vi "3 Mirrors Convert to Volts.vi"(0 "Global Rectangle":i32[](array[numeric]), 2 "Scan Freq (Hz)":dbl, 5 "X Center":dbl, 7 "Y Center":dbl, 9 "M1 Volts Per Px":dbl, 11 "M2 Volts Per Px":dbl) -> (8 "Voltage Data":T1)   [LabVIEW 2020]
uses:
  3 Mirror Scan Type Defs/3 Mirror Scan ROI Voltage Data.ctl
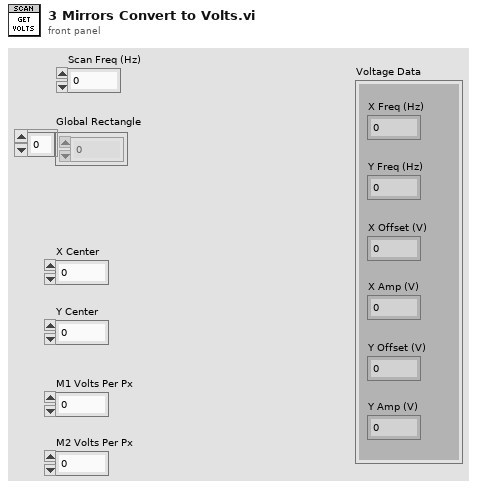
[diagram p1: front panel]
types:
  T1 = typedef "3 Mirror Scan ROI Voltage Data.ctl" = cluster{"X Freq (Hz)":dbl, "Y Freq (Hz)":dbl, "X Offset (V)":dbl, "X Amp (V)":dbl, "Y Offset (V)":dbl, "Y Amp (V)":dbl}
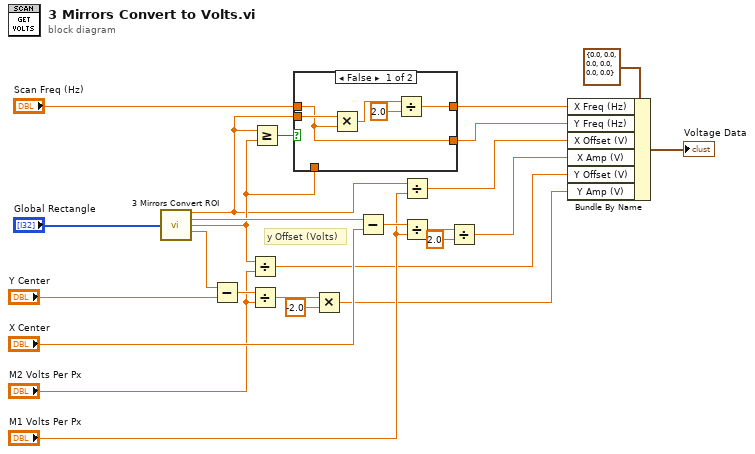
[diagram p0: block diagram]
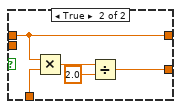
[diagram p2: hidden frame]
diagram:
  # "y Offset (Volts)"
  n1 = call "3 Mirrors Convert ROI.vi"("Global Rectangle"="Global Rectangle") -> ("X Width (px)"=w15:dbl, "X Center (px)"=w25:dbl, "Y Width (px)"=w16:dbl, "Y Center (px)"=w24:dbl)  [unwired: 11 in]
  n2 = Subtract(x=w24, y="Y Center") -> (x-y=w22:dbl)
  n3 = Divide(x=w16, y="M2 Volts Per Px") -> (x/y=w3:dbl)
  n4 = Divide(x=w22, y="M2 Volts Per Px") -> (x/y=w19:dbl)
  n5 = Greater Or Equal?(x=w15, y=w16) -> (x >= y?=w17:bool)
  n6 = case shown="False" w17 {
    tunnel: "Scan Freq (Hz)" -> [w29 w34]
    tunnel: [w26 w34] -> w7
    tunnel: w16 -> [_ w35]
    tunnel: [w29 w31] -> w6
    tunnel: w15 -> [w30 _]
    frame False {
      n7 = Multiply(x=w30, y=w29) -> (x*y=w27:dbl)
      n8 = Divide(x=w27, y=2.0) -> (x/y=w26:dbl)
    }
    frame True {
      n9 = Multiply(x=w34, y=w35) -> (x*y=w32:dbl)
      n10 = Divide(x=w32, y=2.0) -> (x/y=w31:dbl)
    }
  }
  n11 = Multiply(x=w19, y=-2.0) -> (x*y=w2:dbl)
  n12 = Subtract(x=w25, y="X Center") -> (x-y=w23:dbl)
  n13 = Divide(x=w15, y="M1 Volts Per Px") -> (x/y=w5:dbl)
  n14 = Divide(x=w23, y="M1 Volts Per Px") -> (x/y=w21:dbl)
  n15 = Divide(x=w21, y=2.0) -> (x/y=w4:dbl)
  n16 = Bundle By Name(cluster=T1 {"X Freq (Hz)"=0.0, "Y Freq (Hz)"=0.0, "X Offset (V)"=0.0, "X Amp (V)"=0.0, "Y Offset (V)"=0.0, "Y Amp (V)"=0.0} ("Axis Voltage Data"), "X Freq (Hz)"=w7, "Y Freq (Hz)"=w6, "X Offset (V)"=w5, "X Amp (V)"=w4, "Y Offset (V)"=w3, "Y Amp (V)"=w2) -> (→"Voltage Data":T1)
